vi "Network_AI_Shared_Variables_v4.vi"(1 "error in (no error)":errorcluster, 2 "AI Scope Data":T1) -> (0 "error out":errorcluster)   [LabVIEW 2012, in "Labview_Networking.lvlib"]
doc: "Uses DataSocket technology to write live images."
uses:
  Labview_Networking.lvlib
  AI_Scope_Data_v4.ctl
  Controls.llb/Controls.lvlib
panel:
  out "Data Size":i32[](array[numeric])
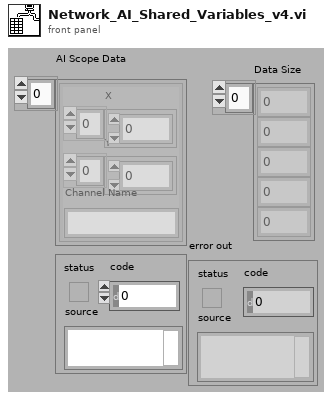
[diagram p1: front panel]
types:
  T1 = typedef "Controls.lvlib/AI_Scope_Data_v4.ctl" = cluster{"X":sgl[], "Y":sgl[], "Channel Name":string}[]
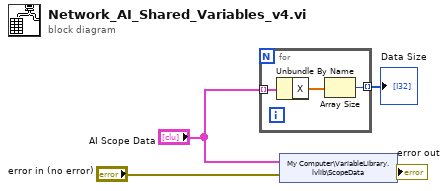
[diagram p0: block diagram]
diagram:
  n1 = for {
    tunnel: "AI Scope Data" -> [w6] mode=indexing
    tunnel: [w7] -> w2 mode=indexing
    n2 = Unbundle By Name(w6) -> ("X"=w5:sgl[])
    n3 = Array Size(array=w5) -> (size(s)=w7:i32)
  }
  "Data Size" <- w2
  n4 = shared-variable "My Computer\\VariableLibrary.lvlib\\ScopeData"("AI Scope Data", error in="error in (no error)") -> (error out=→"error out":errorcluster)
